vi "_Tree_.vi"   [LabVIEW 2020, in "UI_Actor.lvlib"]
uses:
  UI_Actor.lvlib
  UI_Actor/UI_Actor.lvclass
  UI_Actor Messages/UI_AutoRefresh_Init Msg/UI_AutoRefresh_Init Msg.lvclass
  UI_Actor Messages/UI_AutoRefresh_Do Msg/UI_AutoRefresh_Do Msg.lvclass
  UI_Actor Messages/UI_Resize Msg/UI_Resize Msg.lvclass
  UI_Actor Messages/UI_Hide Msg/UI_Hide Msg.lvclass
  UI_Actor Messages/UI_ShowIn_FreeWindow Msg/UI_ShowIn_FreeWindow Msg.lvclass
  UI_Actor Messages/UI_ShowIn_Subpanel Msg/UI_ShowIn_Subpanel Msg.lvclass
  UI_Actor Messages/Ping Tree Msg/Ping Tree Msg.lvclass
  UI_Actor Messages/UI_KBB_Trig Msg/UI_KBB_Trig Msg.lvclass
  UI_Actor/UI_Elmt_Read_MAP.vi
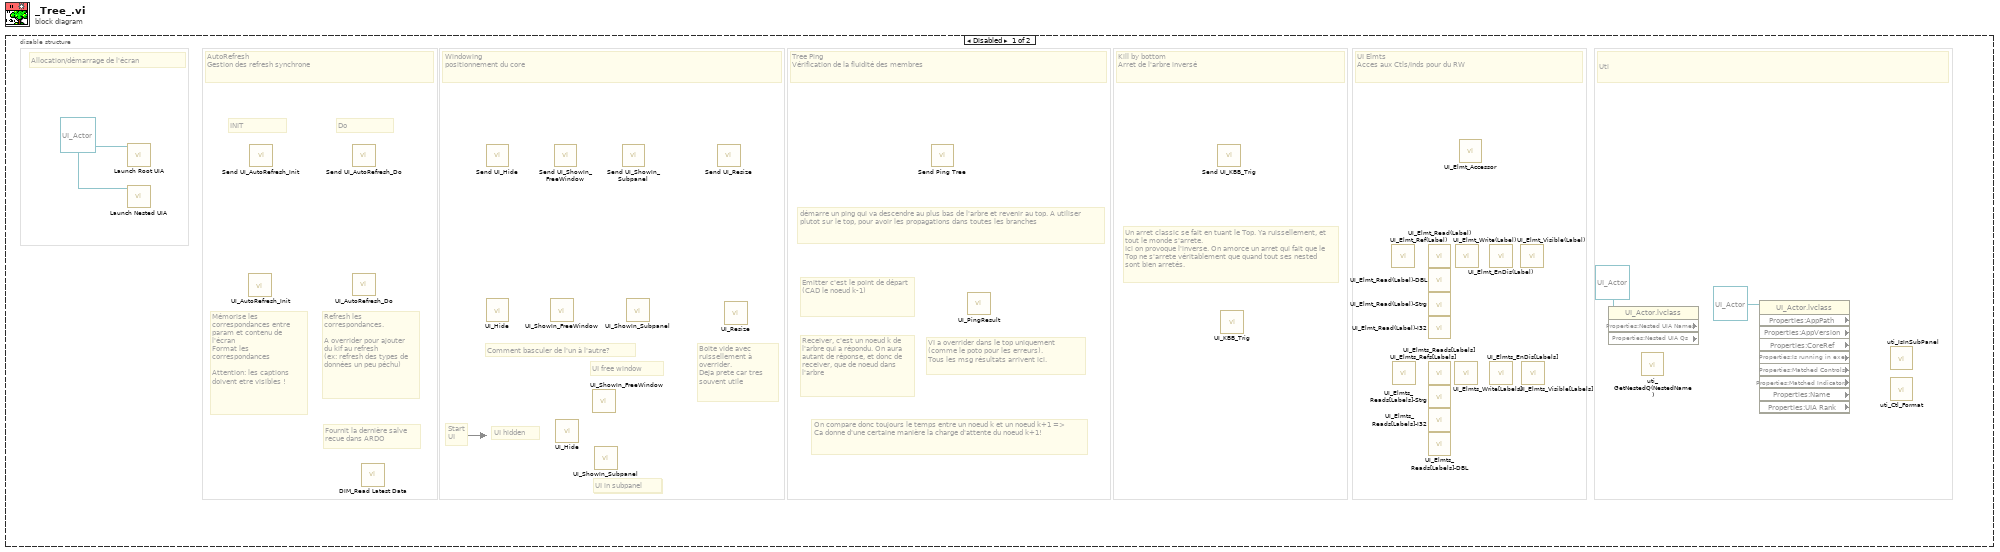
[diagram p0: block diagram]
diagram:
  n1 = disable-structure shown="Disabled" {
    frame Disabled {
      w3 = refnum<class "UI_Actor.lvclass"> refnum ("UI_Actor.lvlib:UI_Actor.lvclass")
      # "Uti"
      # "Fournit la dernière salve recue dans ARDO"
      # "UI Elmts\nAcces aux Ctls/Inds pour du RW"
      # "Un arret classic se fait en tuant le Top. Ya ruissellement, et tout le monde s'arrete.\nIci on provoque l'inverse. On amorce un arret qui fait que le Top ne s'arrete véritablement que quand tout ses nested sont bien arretés."
      # "Kill by bottom\nArret de l'arbre inversé"
      # "Do"
      # "Tree Ping\nVérification de la fluidité des membres"
      # "Boite vide avec ruissellement à overrider.\nDeja prete car tres souvent utile"
      # "UI free window"
      # "UI hidden"
      # "UI in subpanel"
      # "Windowing\npositionnement du core"
      # "INIT"
      # "On compare donc toujours le temps entre un noeud k et un noeud k+1 => Ca donne d'une certaine manière la charge d'attente du noeud k+1!"
      # "Receiver, c'est un noeud k de l'arbre qui a répondu. On aura autant de réponse, et donc de receiver, que de noeud dans l'arbre"
      # "Emitter c'est le point de départ (CAD le noeud k-1)"
      # "VI a overrider dans le top uniquement (comme le poto pour les erreurs).\nTous les msg résultats arrivent ici."
      # "démarre un ping qui va descendre au plus bas de l'arbre et revenir au top. A utiliser plutot sur le top, pour avoir les propagations dans toutes les branches"
      # "Mémorise les correspondances entre param et contenu de l'écran\nFormat les correspondances\n\nAttention: les captions doivent etre visibles !"
      # "AutoRefresh\nGestion des refresh synchrone"
      # "Comment basculer de l'un à l'autre?"
      # "Start\nUI"
      # "UI in subpanel"
      # "UI free window"
      # "UI hidden"
      # "Allocation/démarrage de l'écran"
      # "Refresh les correspondances.\n\nA overrider pour ajouter \ndu kif au refresh\n(ex: refresh des types de données un peu péchu)"
      n2 = call "Launch Root UIA.vi"("UI_Actor in"=w3) -> ()  [unwired: 9 in, 2 out]
      n3 = call "Launch Nested UIA.vi"("Caller UIA in"=w3) -> ()  [unwired: 8 in, 3 out]
      n4 = call-dynamic "UI_AutoRefresh_Init.vi"() -> ()  [unwired: 10 in, 2 out]
      n5 = call "Send UI_AutoRefresh_Init.vi"() -> ()  [unwired: 10 in, 2 out]
      n6 = call "Send UI_AutoRefresh_Do.vi"() -> ()  [unwired: 10 in, 2 out]
      n7 = call-dynamic "UI_AutoRefresh_Do.vi"() -> ()  [unwired: 10 in, 2 out]
      n8 = call "DIM_Read Latest Data.vi"() -> ()  [unwired: 9 in, 3 out]
      n9 = call "Send UI_Hide.vi"() -> ()  [unwired: 10 in, 2 out]
      n10 = call-dynamic "UI_Hide.vi"() -> ()  [unwired: 10 in, 2 out]
      n11 = call-dynamic "UI_ShowIn_FreeWindow.vi"() -> ()  [unwired: 10 in, 2 out]
      n12 = call "Send UI_ShowIn_FreeWindow.vi"() -> ()  [unwired: 10 in, 2 out]
      n13 = call-dynamic "UI_Hide.vi"() -> ()  [unwired: 10 in, 2 out]
      n14 = call-dynamic "UI_ShowIn_FreeWindow.vi"() -> ()  [unwired: 10 in, 2 out]
      n15 = call-dynamic "UI_ShowIn_Subpanel.vi"() -> ()  [unwired: 10 in, 2 out]
      n16 = call "Send UI_ShowIn_Subpanel.vi"() -> ()  [unwired: 10 in, 2 out]
      n17 = call-dynamic "UI_ShowIn_Subpanel.vi"() -> ()  [unwired: 10 in, 2 out]
      n18 = call "Send UI_Resize.vi"() -> ()  [unwired: 10 in, 2 out]
      n19 = call-dynamic "UI_Resize.vi"() -> ()  [unwired: 10 in, 2 out]
      n20 = call "Send Ping Tree.vi"() -> ()  [unwired: 10 in, 2 out]
      n21 = call-dynamic "UI_PingResult.vi"() -> ()  [unwired: 10 in, 2 out]
      n22 = call "Send UI_KBB_Trig.vi"() -> ()  [unwired: 10 in, 2 out]
      n23 = call-dynamic "UI_KBB_Trig.vi"() -> ()  [unwired: 10 in, 2 out]
      n24 = call "UI_Elmt_Ref(Label).vi"() -> ()  [unwired: 8 in, 4 out]
      n25 = call "UI_Elmts_Refs[Labels].vi"() -> ()  [unwired: 8 in, 4 out]
      n26 = call "UI_Elmt_Read(Label).vi"() -> ()  [unwired: 8 in, 4 out]
      n27 = call "UI_Elmt_Read(Label)-DBL.vi"() -> ()  [unwired: 8 in, 4 out]
      n28 = call "UI_Elmt_Read(Label)-Strg.vi"() -> ()  [unwired: 8 in, 4 out]
      n29 = call "UI_Elmt_Read(Label)-I32.vi"() -> ()  [unwired: 8 in, 4 out]
      n30 = call "UI_Elmts_Reads[Labels].vi"() -> ()  [unwired: 8 in, 4 out]
      n31 = call "UI_Elmts_Reads[Labels]-Strg.vi"() -> ()  [unwired: 8 in, 4 out]
      n32 = call "UI_Elmts_Reads[Labels]-I32.vi"() -> ()  [unwired: 8 in, 4 out]
      n33 = call "UI_Elmts_Reads[Labels]-DBL.vi"() -> ()  [unwired: 8 in, 4 out]
      n34 = call "UI_Elmts_Write[Labels].vi"() -> ()  [unwired: 9 in, 3 out]
      n35 = call "UI_Elmt_Write(Label).vi"() -> ()  [unwired: 9 in, 3 out]
      n36 = call-poly "UI_Elmt_Accessor.vi"() -> ()  [unwired: 9 in, 3 out]
      n37 = call "UI_Elmt_EnDis(Label).vi"() -> ()  [unwired: 9 in, 3 out]
      n38 = call "UI_Elmts_EnDis[Labels].vi"() -> ()  [unwired: 9 in, 3 out]
      n39 = call "UI_Elmt_Visible(Label).vi"() -> ()  [unwired: 9 in, 3 out]
      n40 = call "UI_Elmts_Visible[Labels].vi"() -> ()  [unwired: 9 in, 3 out]
      n41 = property class="UI_Actor.lvclass" props=["Properties:Nested UIA Names", "Properties:Nested UIA Qs"](reference=refnum<class "UI_Actor.lvclass"> refnum ("UI_Actor in")) -> ()  [unwired: 1 in, 4 out]
      n42 = call "uti_GetNestedQ(NestedName).vi"() -> ()  [unwired: 9 in, 3 out]
      n43 = property class="UI_Actor.lvclass" props=["Properties:AppPath", "Properties:AppVersion", "Properties:CoreRef", "Properties:Is running in exe", "Properties:Matched Controls", "Properties:Matched Indicators", "Properties:Name", "Properties:UIA Rank"](reference=refnum<class "UI_Actor.lvclass"> refnum ("UI_Actor in")) -> ()  [unwired: 1 in, 10 out]
      n44 = call "uti_IsInSubPanel.vi"() -> ()  [unwired: 9 in, 3 out]
      n45 = call "uti_Ctl_Format.vi"() -> ()  [unwired: 10 in, 2 out]
    }
    frame Enabled {
    }
  }
